vi "Ballard - Arinc-429 - Load Parameters File.vi"(8 "error in (no error)":errorcluster, 11 "Node Ptr":u64 format="%.0x") -> (0 "error out":errorcluster)   [LabVIEW 2019, in "Ballard Arinc-429 System Explorer.lvlib"]
uses:
  Ballard Arinc-429 System Explorer.lvlib
  SubVIs/Create Sysdef Tree from Parameters Clusters.vi
  SubVIs/Create Sysdef Tree from Parameters Clusters_Find Label Refs.vi
  SubVIs/Create Sysdef Tree from Parameters Clusters_Find Channel Ref.vi
  Shared/Controls and Global/Global.vi
  <vilib>/NI VeriStand/Custom Device API/Get Item Property (Path).vi
  SubVIs/Parse Parameters File/Read_XML_Parameters File_002.vi
  <vilib>/NI VeriStand/Custom Device API/NI VeriStand - Enable System Explorer Update Buffer.vi
  <vilib>/NI VeriStand/Custom Device Tools/Custom Device Utility Library/NI VeriStand - Search for Item.vi
  <vilib>/NI VeriStand/Custom Device Tools/Custom Device Utility Library/NI VeriStand - Search for Item by GUID.vi
  <vilib>/NI VeriStand/Custom Device Tools/Custom Device Utility Library/NI VeriStand - Search for All Items by GUID.vi
  <vilib>/NI VeriStand/Custom Device API/Get Item Property (U16).vi
  <vilib>/NI VeriStand/Custom Device API/NI VeriStand - Get Item Children.vi
  <vilib>/NI VeriStand/Custom Device API/Get Item Property (U32).vi
  <vilib>/NI VeriStand/Custom Device API/Get Item Property (Boolean).vi
  <vilib>/NI VeriStand/Custom Device API/NI VeriStand - Get Item Data.vi
  <vilib>/NI VeriStand/Custom Device Tools/Custom Device Utility Library/NI VeriStand - Get All Channels.vi
  <vilib>/NI VeriStand/Custom Device API/NI VeriStand - Remove Custom Device Item.vi
  SubVIs/AddParamChannels.vi
  <vilib>/NI VeriStand/Custom Device API/NI VeriStand - Commit System Explorer Update Buffer.vi
  <vilib>/NI VeriStand/Custom Device API/Set Item Property (String).vi
  <vilib>/NI VeriStand/Custom Device API/Set Item Property (Path).vi
  <vilib>/NI VeriStand/Custom Device API/Custom Device API.lvlib
  Shared/Ballard Arinc-429 Shared.lvlib
  <vilib>/NI VeriStand/Custom Device Tools/Custom Device Utility Library/Custom Device Utility Library.lvlib
panel:
  in  "Tag":string
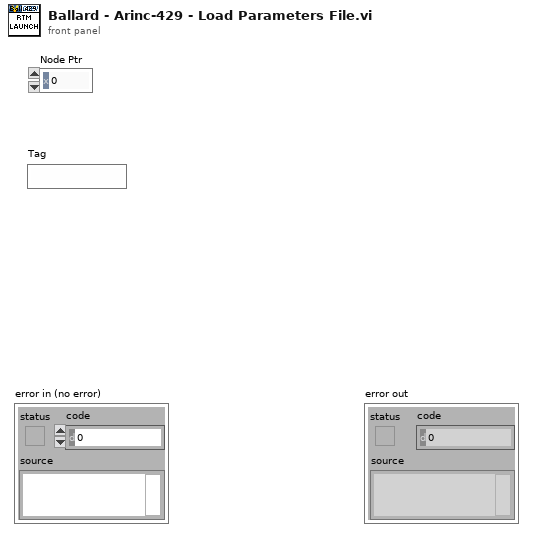
[diagram p1: front panel]
types:
  T1 = typedef "Custom Device API.lvlib/Custom Device Item Ref.ctl" = u64
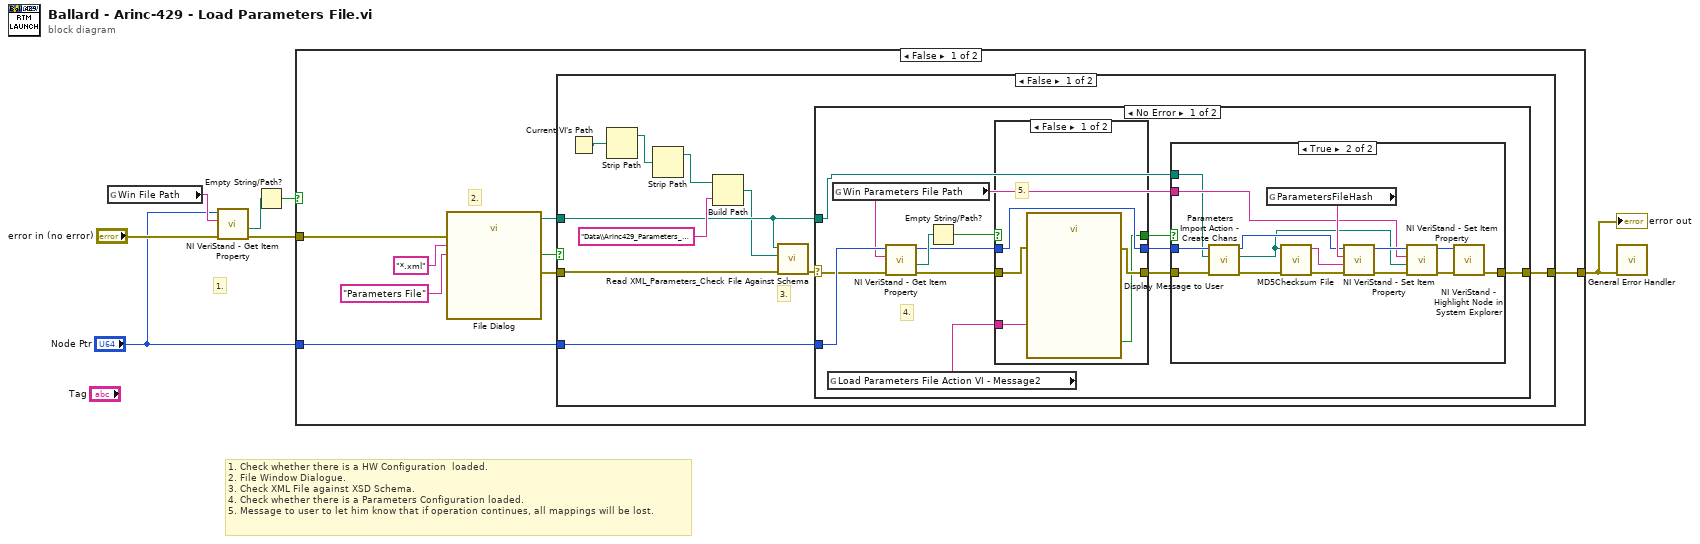
[diagram p0: block diagram]
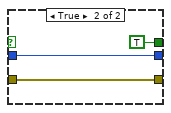
[diagram p2: hidden frame]
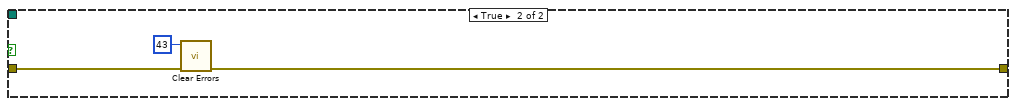
[diagram p5: hidden frame]
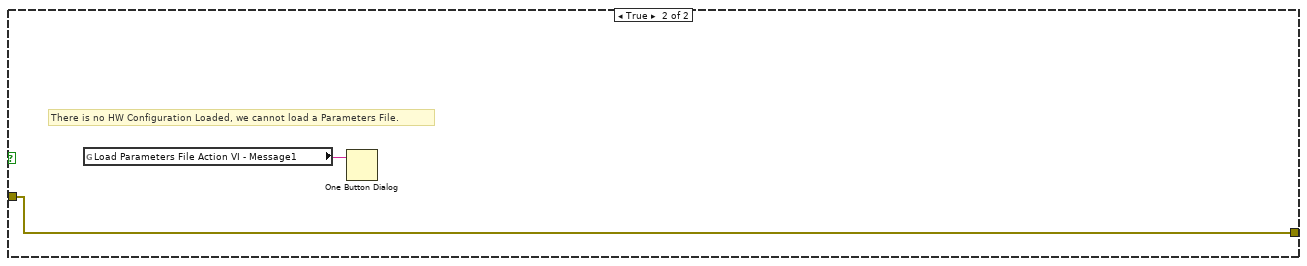
[diagram p6: hidden frame]
diagram:
  # "1. Check whether there is a HW Configuration  loaded.\n2. File Window Dialogue.\n3. Check XML File against XSD Schema.\n4. Check whether there is a Parameters Configuration loaded.\n5. Message to user to let him know that if operation continues, all mappings will be lost."
  # "1."
  n1 = global read "Global.vi" "Win File Path"() -> (w6:string)
  n2 = call-poly <vilib>:"NI VeriStand - Get Item Property.vi"("error in (no error)"="error in (no error)", "Property Name"=w6, "Item Ref in"="Node Ptr") -> ("error out"=w2:errorcluster, "Value"=w5:path)  [unwired: 5 in, 2 out]
  n3 = Empty String/Path?(string/path=w5) -> (empty?=w1:bool)
  n4 = case shown="False" w1 {
    tunnel: [w15 w67] -> w7
    tunnel: "Node Ptr" -> [w9 _]
    tunnel: w2 -> [w8 w67]
    frame False {
      # "2."
      n5 = call "File Dialog"("error in"=w8, "pattern (all files)"="*.xml", "pattern label"="Parameters File") -> ("selected path"=w10:path, "cancelled"=w12:bool, "error out"=w11:errorcluster)  [unwired: 9 in, 1 out]
      n6 = case shown="False" w12 {
        tunnel: [w25 w65] -> w15
        tunnel: w11 -> [w22 w66]
        tunnel: w9 -> [w24 _]
        tunnel: w10 -> [w17 _]
        frame False {
          # "3."
          n7 = Current VI's Path() -> (path=w19:path)
          n8 = Strip Path(path=w19) -> (stripped path=w20:path)  [unwired: 1 out]
          n9 = Strip Path(path=w20) -> (stripped path=w21:path)  [unwired: 1 out]
          n10 = Build Path(base path=w21, name or relative path="Data\\Arinc429_Parameters_XML_Schema.xsd") -> (appended path=w16:path)
          n11 = call "Read XML_Parameters_Check File Against Schema.vi"("error in (no error)"=w22, "XML Schema File Path"=w16, "XML Configuration File Path"=w17) -> ("error IO"=w23:errorcluster)  [unwired: 7 in, 1 out]
          n12 = case shown="No Error" w23 {
            selector: w23 -> [w35 w63]
            tunnel: [w38 w63] -> w25
            tunnel: w24 -> [w37 _]
            tunnel: w17 -> [w27 _]
            frame No Error {
              # "4."
              n13 = global read "Global.vi" "Load Parameters File Action VI - Message2"() -> (w26:string)
              n14 = global read "Global.vi" "Win Parameters File Path"() -> (w34:string)
              n15 = call-poly <vilib>:"NI VeriStand - Get Item Property.vi"("error in (no error)"=w35, "Property Name"=w34, "Item Ref in"=w37) -> ("error out"=w32:errorcluster, "Value"=w36:path, "Item Ref out"=w31:T1)  [unwired: 5 in, 1 out]
              n16 = Empty String/Path?(string/path=w36) -> (empty?=w33:bool)
              n17 = case shown="False" w33 {
                tunnel: w32 -> [w42 w45]
                tunnel: w31 -> [w43 w44]
                tunnel: [w40 TRUE] -> w30
                tunnel: [w41 w45] -> w29
                tunnel: [w43 w44] -> w28
                tunnel: w26 -> [w39 _]
                frame False {
                  # "5."
                  n18 = call "Display Message to User"("error in (no error)"=w42, "Message"=w39) -> ("error out"=w41:errorcluster, "OK"=w40:bool)  [unwired: 8 in]
                }
                frame True {
                }
              }
              n19 = case shown="True" w30 {
                tunnel: [w47 w62] -> w38
                tunnel: w34 -> [_ w54]
                tunnel: w29 -> [w47 w52]
                tunnel: w28 -> [_ w53]
                tunnel: w27 -> [_ w49]
                frame False {
                }
                frame True {
                  n20 = call "Parameters Import Action - Create Chans.vi"("error in (no error)"=w52, "selected path"=w49, "Node Ptr"=w53) -> ("error out"=w50:errorcluster, "selected path out"=w48:path, "Node Ptr dup"=w51:u64)  [unwired: 6 in]
                  n21 = global read "Global.vi" "ParametersFileHash"() -> (w61:string)
                  n22 = call <vilib>:"MD5Checksum File.vi"("error in (no error)"=w50, "Path"=w48) -> ("error out"=w56:errorcluster, "MD5 message-digest"=w55:string)  [unwired: 8 in]
                  n23 = call-poly <vilib>:"NI VeriStand - Set Item Property.vi"("error in (no error)"=w56, "Value"=w55, "Property Name"=w61, "Item Ref in"=w51) -> ("error out"=w57:errorcluster, "Item Ref out"=w58:T1)  [unwired: 5 in, 1 out]
                  n24 = call-poly <vilib>:"NI VeriStand - Set Item Property.vi"("error in (no error)"=w57, "Value"=w48, "Property Name"=w54, "Item Ref in"=w58) -> ("error out"=w60:errorcluster, "Item Ref out"=w59:T1)  [unwired: 5 in, 1 out]
                  n25 = call <vilib>:"NI VeriStand - Highlight Node in System Explorer.vi"("error in (no error)"=w60, "Item Ref in"=w59) -> ("error out"=w62:errorcluster)  [unwired: 8 in, 1 out]
                }
              }
            }
            frame Error {
            }
          }
        }
        frame True {
          n26 = call <vilib>:"Clear Errors.vi"("error in (no error)"=w66, "specific error code to clear (0: all)"=43) -> ("error out"=w65:errorcluster)  [unwired: 4 in, 1 out]
        }
      }
    }
    frame True {
      # "There is no HW Configuration Loaded, we cannot load a Parameters File."
      n27 = global read "Global.vi" "Load Parameters File Action VI - Message1"() -> (w68:string)
      n28 = One Button Dialog(message=w68) -> ()  [unwired: 1 in, 1 out]
    }
  }
  "error out" <- w7
  n29 = call <vilib>:"General Error Handler.vi"("error in (no error)"=w7) -> ()  [unwired: 10 in, 5 out]
